vi "Time SET.vi"(8 "Err_IN":errorcluster caption="에러 상수") -> (0 "Err_Out":errorcluster caption="에러 상수", 3 "배열":i32[](array[numeric]))   [LabVIEW 2023]
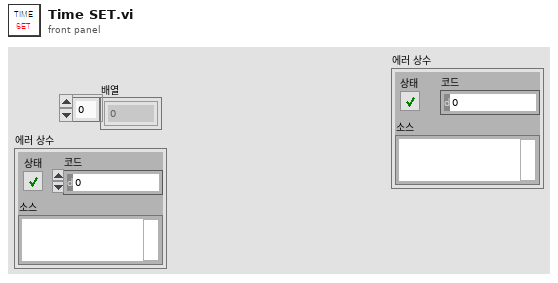
[diagram p1: front panel]
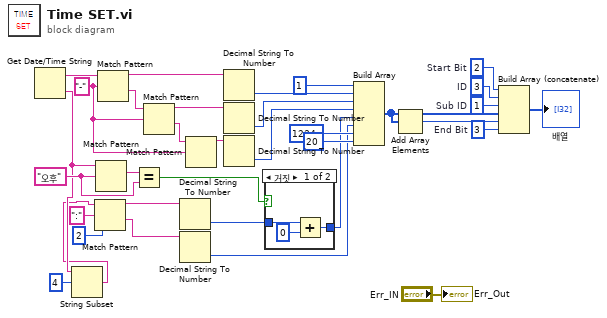
[diagram p0: block diagram]
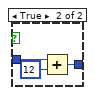
[diagram p2: hidden frame]
diagram:
  w33 = 3  # End Bit
  w30 = 1  # Sub ID
  w29 = 3  # ID
  w28 = 2  # Start Bit
  w18 = "오후" ("정규식")
  w10 = "-" ("정규식")
  n1 = Get Date/Time String() -> (date string=w7:string, time string=w3:string)  [unwired: 3 in]
  n2 = String Subset(string=w3, offset (0)=4 ("오프셋(0)")) -> (substring=w1:string)  [unwired: 1 in]
  n3 = Match Pattern(string=w1, regular expression=":" ("정규식"), offset (0)=2 ("오프셋(0)")) -> (before substring=w20:string, after substring=w21:string)  [unwired: 2 out]
  n4 = Match Pattern(string=w3, regular expression=w18) -> (match substring=w17:string)  [unwired: 1 in, 3 out]
  n5 = Match Pattern(string=w7, regular expression=w10) -> (before substring=w8:string, after substring=w5:string)  [unwired: 1 in, 2 out]
  n6 = Equal?(x=w17, y=w18) -> (x = y?=w23:bool)
  n7 = Match Pattern(string=w5, regular expression=w10) -> (before substring=w11:string, after substring=w9:string)  [unwired: 1 in, 2 out]
  n8 = Decimal String To Number(string=w20) -> (number=w22:i32)  [unwired: 2 in, 1 out]
  n9 = Decimal String To Number(string=w21) -> (number=w25:i32)  [unwired: 2 in, 1 out]
  n10 = Match Pattern(string=w9, regular expression=w10) -> (before substring=w12:string)  [unwired: 1 in, 3 out]
  n11 = Decimal String To Number(string=w8) -> (number=w14:i32)  [unwired: 2 in, 1 out]
  n12 = Decimal String To Number(string=w11) -> (number=w15:i32)  [unwired: 2 in, 1 out]
  n13 = Decimal String To Number(string=w12) -> (number=w16:i32)  [unwired: 2 in, 1 out]
  n14 = case shown="거짓" w23 {
    tunnel: w22 -> [w37 w40]
    tunnel: [w35 w38] -> w24
    frame False {
      n15 = Add(x=w37, y=0) -> (x+y=w35:i32)
    }
    frame True {
      n16 = Add(x=w40, y=12) -> (x+y=w38:i32)
    }
  }
  n17 = Build Array(1 ("원소"), w14, w15, w16, w24, w25, 1234 ("원소"), 20 ("원소")) -> (w32:i32[])
  n18 = Add Array Elements(numeric array=w32) -> (sum=w31:i32)
  n19 = Build Array (concatenate)(w28, w29, w30, w32, w31, w33) -> (→"배열":i32[])
  "Err_Out" <- "Err_IN"
